vi "XY Graph Get Convolution Step.vi"(6 "Reference Decay":cluster{"t Array":dbl[], "I Array":dbl[]}, 7 "Time Step":T1, 8 "Error In":errorcluster, 9 "# Plots":i32, 10 "Selected Plot":i32, 11 "XYGraph in":T2) -> (0 "Error Out":errorcluster, 3 "Step":dbl[unit])   [LabVIEW 2021, in "XY Graph Add-Ons.lvlib"]
uses:
  XY Graph Add-Ons.lvlib
  XY Graph Refnum.ctl
  XY Graph Convolution Step Type.ctl
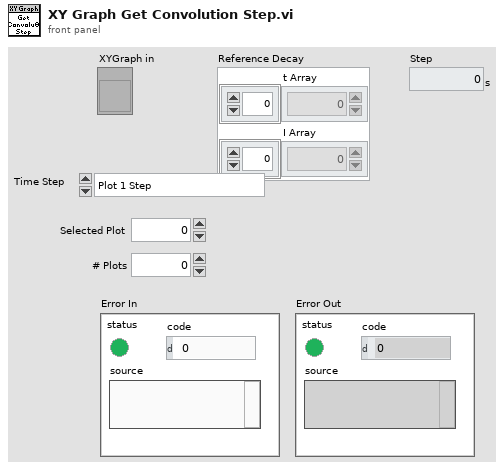
[diagram p1: front panel]
types:
  T1 = typedef "XY Graph Add-Ons.lvlib/XY Graph Convolution Step Type.ctl" = enum16{"Plot 1 Step", "Plot 2 Step", "User Defined"}
  T2 = typedef "XY Graph Add-Ons.lvlib/XY Graph Refnum.ctl" = refnum<vi>
  T3 = typedef "XY Graph Add-Ons.lvlib/XY Plot Data.ctl" = cluster{"X Array":dbl[], "Y Array":dbl[]}
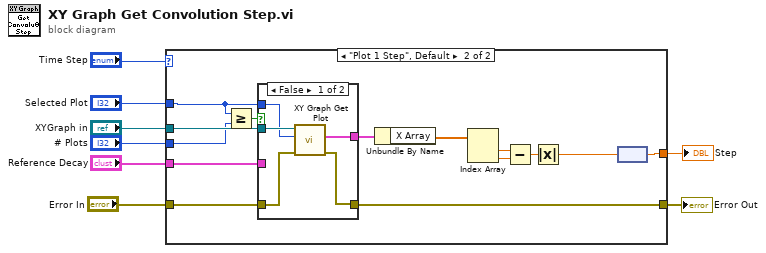
[diagram p0: block diagram]
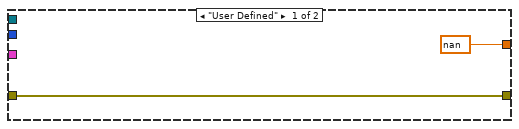
[diagram p2: hidden frame]
diagram:
  n1 = case shown="\"Plot 1 Step\", Default" "Time Step" {
    tunnel: [dbl[unit] nan ("Value (Signaling)") w15] -> w4
    tunnel: "XYGraph in" -> [_ w24]
    tunnel: "# Plots" -> [_ w23]
    tunnel: "Reference Decay" -> [_ w21]
    tunnel: "Selected Plot" -> [_ w14]
    tunnel: "Error In" -> [w10 w13]
    tunnel: [w10 w12] -> w1
    frame "User Defined" {
    }
    frame "Plot 1 Step", Default {
      n2 = Greater Or Equal?(x=w14, y=w23) -> (x >= y?=w22:bool)
      n3 = case shown="False" w22 {
        tunnel: w24 -> [w29 _]
        tunnel: w14 -> [w25 _]
        tunnel: [w28 w31] -> w20
        tunnel: w21 -> [_ w31]
        tunnel: w13 -> [w27 w30]
        tunnel: [w26 w30] -> w12
        frame False {
          n4 = call "XY Graph Get Plot.vi"("error in (no error)"=w27, "Plot Index (-1: last)"=w25, "XYGraph in"=w29) -> ("error out"=w26:errorcluster, "Plot Data"=w28:T3)  [unwired: 4 in, 3 out]
        }
        frame True {
        }
      }
      n5 = Unbundle By Name(w20) -> ("X Array"=w19:dbl[])
      n6 = Index Array(array=w19) -> (element #1=w18:dbl, element #2=w17:dbl)  [unwired: 2 in]
      n7 = Subtract(x=w18, y=w17) -> (x-y=w16:dbl)
      n8 = Absolute Value(x=w16) -> (abs(x)=w11:dbl)
      n9 = node(w11) -> (w15:dbl[unit])
    }
  }
  "Step" <- w4
  "Error Out" <- w1
